vi "destroy IMAQ references.vi"(8 "error in (no error)":errorcluster, 11 "Cascade in":refnum<class "Cascade.lvclass">) -> (0 "error out":errorcluster, 3 "Cascade out":refnum<class "Cascade.lvclass">)   [LabVIEW 2012, in "Cascade.lvclass"]
uses:
  Cascade.lvclass
  Cascade.lvclass/Cascade.ctl
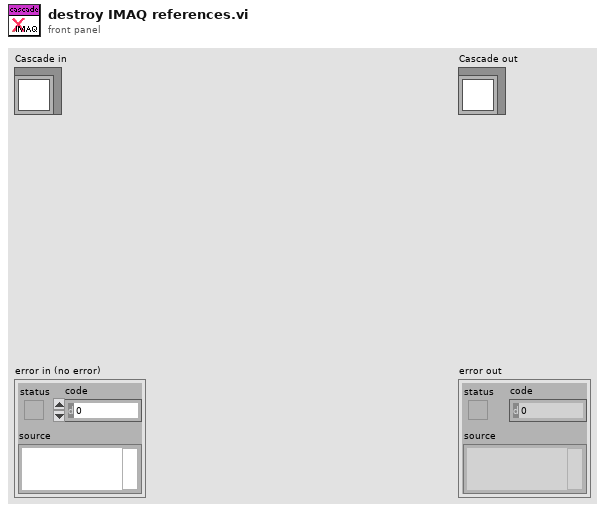
[diagram p1: front panel]
types:
  T1 = typedef "IMAQ Image.ctl" = refnum<image>
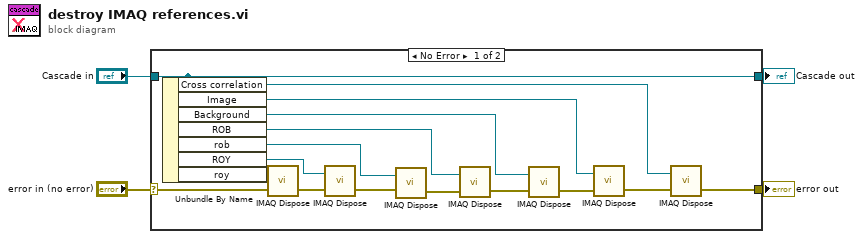
[diagram p0: block diagram]
diagram:
  n1 = case shown="No Error" "error in (no error)" {
    selector: "error in (no error)" -> [w20 w22]
    tunnel: [w6 w22] -> w3
    tunnel: [w14 w21] -> w1
    tunnel: "Cascade in" -> [w14 w21]
    frame No Error {
      n2 = Unbundle By Name(w14) -> ("Cross correlation"=w5:T1, "Image"=w8:T1, "Background"=w9:T1, "ROB"=w10:T1, "rob"=w11:T1, "ROY"=w12:T1, "roy"=w13:T1)
      n3 = call "IMAQ Dispose"("Image"=w13, "error in (no error)"=w20) -> ("error out"=w19:errorcluster)  [unwired: 4 in]
      n4 = call "IMAQ Dispose"("Image"=w12, "error in (no error)"=w19) -> ("error out"=w18:errorcluster)  [unwired: 4 in]
      n5 = call "IMAQ Dispose"("Image"=w11, "error in (no error)"=w18) -> ("error out"=w17:errorcluster)  [unwired: 4 in]
      n6 = call "IMAQ Dispose"("Image"=w10, "error in (no error)"=w17) -> ("error out"=w16:errorcluster)  [unwired: 4 in]
      n7 = call "IMAQ Dispose"("Image"=w9, "error in (no error)"=w16) -> ("error out"=w15:errorcluster)  [unwired: 4 in]
      n8 = call "IMAQ Dispose"("Image"=w8, "error in (no error)"=w15) -> ("error out"=w7:errorcluster)  [unwired: 4 in]
      n9 = call "IMAQ Dispose"("Image"=w5, "error in (no error)"=w7) -> ("error out"=w6:errorcluster)  [unwired: 4 in]
    }
    frame Error {
    }
  }
  "error out" <- w3
  "Cascade out" <- w1
